vi "Friction Voltage.vi"(0 "Joint Coordinate (rad)":dbl[](array[numeric]), 11 "Raw Voltage Command (volt)":dbl[](array[numeric])) -> (8 "Friction Voltage":dbl)   [LabVIEW 2017]
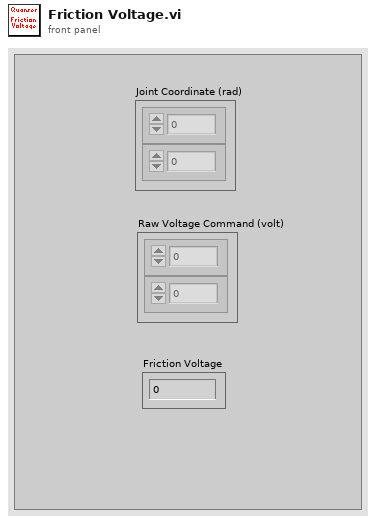
[diagram p1: front panel]
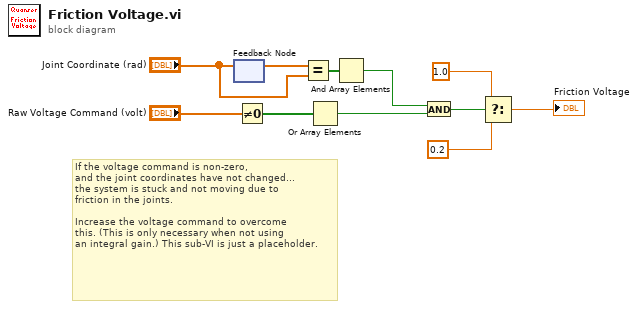
[diagram p0: block diagram]
diagram:
  # "If the voltage command is non-zero, \nand the joint coordinates have not changed...\nthe system is stuck and not moving due to \nfriction in the joints. \n\nIncrease the voltage command to overcome \nthis. (This is only necessary when not using \nan integral gain.) This sub-VI is just a placeholder."
  n1 = feedback #1() -> (w8:dbl[])  [unwired: 1 in]
  n2 = feedback-in #1("Joint Coordinate (rad)") -> ()
  n3 = Not Equal To 0?(x="Raw Voltage Command (volt)") -> (x != 0?=w3:bool[])
  n4 = Equal?(x=w8, y="Joint Coordinate (rad)") -> (x = y?=w5:bool[])
  n5 = Or Array Elements(Boolean array=w3) -> (logical OR=w2:bool)
  n6 = And Array Elements(Boolean array=w5) -> (logical AND=w4:bool)
  n7 = And(x=w4, y=w2) -> (x .and. y?=w1:bool)
  n8 = Select(t=1.0, s=w1, f=0.2) -> (s? t:f=→"Friction Voltage":dbl)
